vi "SubpanelPaths.vi"(8 "error in (no error)":errorcluster, 11 "SMO.UI.MAUI in":refnum<class "SMO.UI.MAUI.lvclass">) -> (0 "error out":errorcluster, 1 "Default?":bool, 2 "Subpanels":path[](array[path]), 3 "SMO.UI.MAUI out":refnum<class "SMO.UI.MAUI.lvclass">)   [LabVIEW 2020, in "SMO.UI.MAUI.lvclass"]
uses:
  SMO.UI.MAUI.lvclass
  <vilib>/addons/_JKI.lib/Serialization/JSON/JKI JSON Serialization.lvlib
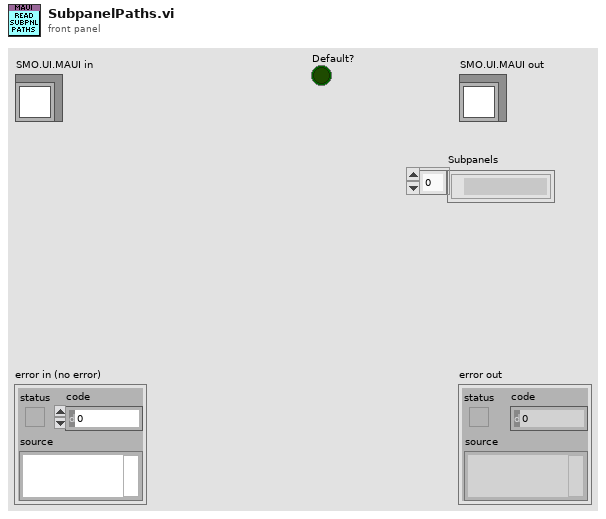
[diagram p1: front panel]
types:
  T1 = enum16{"open", "replace", "create", "open or create", "replace or create", "replace or create with confirmation"}
  T2 = typedef "SMO.UI.MAUI.lvclass/DefaultConfiguration.ctl" = cluster{"Default Subpanel Path":string}
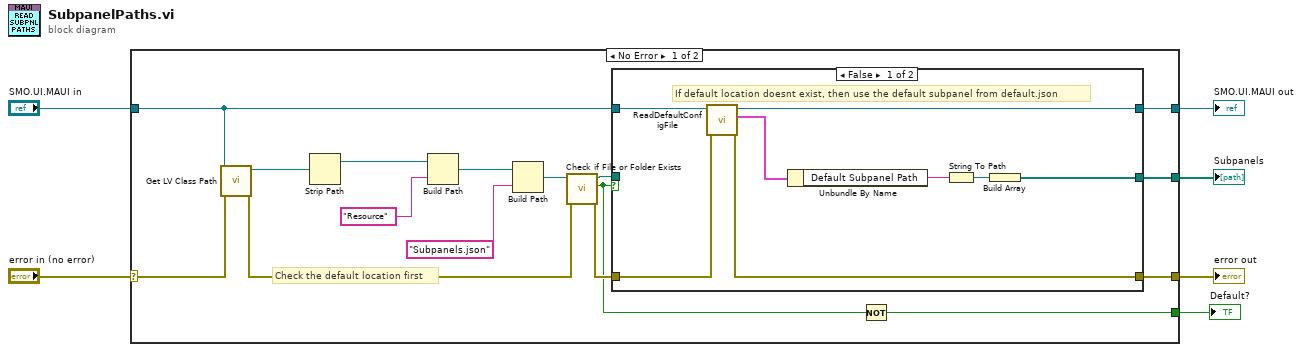
[diagram p0: block diagram]
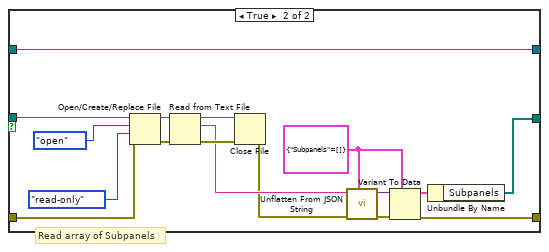
[diagram p2: hidden frame]
diagram:
  n1 = case shown="No Error" "error in (no error)" {
    selector: "error in (no error)" -> [w18 w49]
    tunnel: [w14 w49] -> w5
    tunnel: [w11 w48] -> w3
    tunnel: "SMO.UI.MAUI in" -> [w9 w48]
    tunnel: [w12 _] -> w2
    tunnel: [w7 _] -> w1
    frame No Error {
      # "Check the default location first"
      n2 = call <vilib>:"Get LV Class Path.vi"("error in (no error)"=w18, "object"=w9) -> ("error out"=w17:errorcluster, "class path"=w10:path)  [unwired: 8 in]
      n3 = Strip Path(path=w10) -> (stripped path=w21:path)  [unwired: 1 out]
      n4 = Build Path(base path=w21, name or relative path="Resource") -> (appended path=w19:path)
      n5 = Build Path(base path=w19, name or relative path="Subpanels.json") -> (appended path=w13:path)
      n6 = call <vilib>:"Check if File or Folder Exists.vi"("error in (no error)"=w17, "path"=w13) -> ("error out"=w15:errorcluster, "file or folder exists?"=w8:bool, "dup path"=w16:path)  [unwired: 7 in]
      n7 = case shown="False" w8 {
        tunnel: w16 -> [_ w45]
        tunnel: w15 -> [w27 w31]
        tunnel: [w26 w37] -> w14
        tunnel: [w23 w33] -> w12
        tunnel: [w28 w32] -> w11
        tunnel: w9 -> [w29 w32]
        frame False {
          # "If default location doesnt exist, then use the default subpanel from default.json"
          n8 = call "ReadDefaultConfigFile.vi"("error in (no error)"=w27, "SMO.UI.MAUI in"=w29) -> ("error out"=w26:errorcluster, "Default Data"=w25:T2, "SMO.UI.MAUI out"=w28:refnum<class "SMO.UI.MAUI.lvclass">)  [unwired: 7 in]
          n9 = Unbundle By Name(w25) -> ("Default Subpanel Path"=w24:string)
          n10 = String To Path(string=w24) -> (path=w30:path)
          n11 = Build Array(w30) -> (w23:path[])
        }
        frame True {
          w36 = cluster{"Subpanels":path[]} {"Subpanels"=[]}
          # "Read array of Subpanels"
          n12 = Open/Create/Replace File(file path (use dialog)=w45, error in=w31, operation (0:open)=T1."open", access (0:read/write)=enum16{"read/write", "read-only", "write-only"}."read-only") -> (refnum out=w47:refnum<file>, error out=w44:errorcluster)  [unwired: 2 in, 1 out]
          n13 = Read from Text File(file (use dialog)=w47, error in=w44) -> (refnum out=w46:refnum<file>, text=w40:string, error out=w43:errorcluster)  [unwired: 2 in, 1 out]
          n14 = Close File(refnum=w46, error in=w43) -> (error out=w34:errorcluster)  [unwired: 1 out]
          n15 = call <vilib>:"Unflatten From JSON String.vi"("Type and Defaults"=w36, "error in (no error)"=w34, "JSON String"=w40) -> ("error out"=w38:errorcluster, "Variant"=w39:variant)  [unwired: 7 in]
          n16 = Variant To Data(error in=w38, type=w36, Variant=w39) -> (data=w35:cluster{"Subpanels":path[]}, error out=w37:errorcluster)
          n17 = Unbundle By Name(w35) -> ("Subpanels"=w33:path[])
        }
      }
      n18 = Not(x=w8) -> (.not. x?=w7:bool)
    }
    frame Error {
    }
  }
  "error out" <- w5
  "SMO.UI.MAUI out" <- w3
  "Subpanels" <- w2
  "Default?" <- w1
